vi "servocontrol.vi"() -> ()   [LabVIEW 2021]
uses:
  <vilib>/Utility/error.llb/DialogType.ctl
  <vilib>/DAQmx/write.llb/DAQmx Write (Counter Time 1Chan 1Samp).vi
  <vilib>/DAQmx/create/channels.llb/DAQmx Create Channel (CO-Pulse Generation-Time).vi
  <vilib>/DAQmx/configure/timing.llb/DAQmx Timing (Implicit).vi
  <vilib>/DAQmx/miscellaneous.llb/DAQmx Fill In Error Info.vi
panel:
  in  "RC Servo PWM":dbl(knob)=0.001500001840510888 scale=0.001..0.002 scale format="%#_4g"
  in  "stop":bool
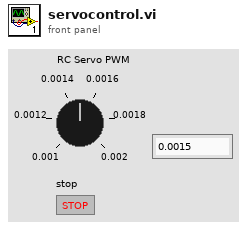
[diagram p1: front panel]
types:
  T1 = typedef "DialogType.ctl" = u16
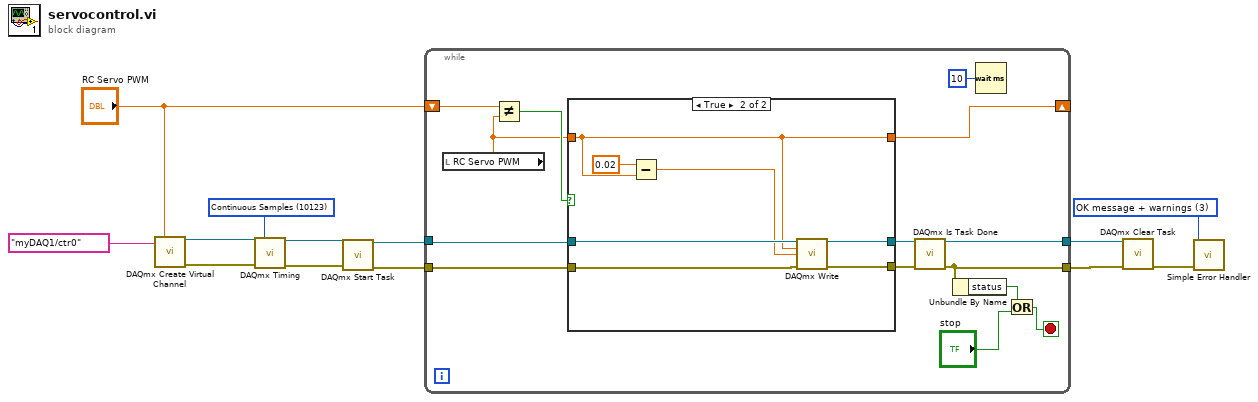
[diagram p0: block diagram]
diagram:
  w2 = T1 3 items=["no dialog", "OK message", "continue or stop message", "OK message + warnings", "continue/stop + warnings"] ("type of dialog (OK msg:1)")
  w9 = 10123 items=["Finite Samples"=10178, "Continuous Samples"=10123, "Hardware Timed Single Point"=12522] ("sample mode")
  n1 = call-poly <vilib>:"DAQmx Create Virtual Channel.vi"("high time"="RC Servo PWM", "counter"=tag "myDAQ1/ctr0") -> ("task out"=w13:refnum<k21>, "error out"=w12:errorcluster)  [unwired: 12 in]
  n2 = call-poly <vilib>:"DAQmx Timing.vi"("task/channels in"=w13, "sample mode"=w9, "error in"=w12) -> ("task out"=w11:refnum<k21>, "error out"=w10:errorcluster)  [unwired: 11 in]
  n3 = call <vilib>:"DAQmx Start Task.vi"("task/channels in"=w11, "error in"=w10) -> ("task out"=w7:refnum<k21>, "error out"=w6:errorcluster)  [unwired: 12 in]
  n4 = while {
    tunnel: w7 -> [w23]
    tunnel: w6 -> [w22]
    tunnel: [w15] -> w5
    tunnel: [w19] -> w4
    shift-right: [w16] -> _
    shift-left: "RC Servo PWM" -> [w25]
    stop <- w18 stop-if-true
    n5 = local read "RC Servo PWM"() -> (w24:dbl)
    n6 = Not Equal?(x=w25, y=w24) -> (x != y?=w26:bool)
    n7 = case shown="True" w26 {
      tunnel: w24 -> [w30 w31]
      tunnel: w23 -> [w29 w37]
      tunnel: w22 -> [w28 w36]
      tunnel: [w29 w35] -> w20
      tunnel: [w28 w34] -> w21
      tunnel: [w30 w31] -> w16
      frame False {
      }
      frame True {
        n8 = Subtract(x=0.02, y=w31) -> (x-y=w32:dbl)
        n9 = call-poly <vilib>:"DAQmx Write.vi"("task/channels in"=w37, "high time"=w31, "low time"=w32, "error in"=w36) -> ("task out"=w35:refnum<k21>, "error out"=w34:errorcluster)  [unwired: 9 in, 1 out]
      }
    }
    n10 = call <vilib>:"DAQmx Is Task Done.vi"("task/channels in"=w20, "error in"=w21) -> ("task out"=w19:refnum<k21>, "error out"=w15:errorcluster)  [unwired: 11 in, 1 out]
    n11 = Unbundle By Name(w15) -> ("status"=w14:bool)
    n12 = Wait (ms)(milliseconds to wait=u32 10) -> ()  [unwired: 1 out]
    n13 = Or(x=w14, y="stop") -> (x .or. y?=w18:bool)
  }
  n14 = call <vilib>:"DAQmx Clear Task.vi"("task in"=w4, "error in"=w5) -> ("error out"=w3:errorcluster)  [unwired: 13 in]
  n15 = call <vilib>:"Simple Error Handler.vi"("type of dialog (OK msg:1)"=w2, "error in (no error)"=w3) -> ()  [unwired: 3 in, 5 out]
